vi "Read Value.vi"(8 "error in (no error)":errorcluster caption="entrée d'erreur (pas d'erreur)", 11 "DAQmxTaskAITension_Emulate en entrée":refnum<class "DAQmxTaskAIVoltage_Emulate.lvclass">) -> (0 "error out":errorcluster caption="sortie d'erreur", 1 "Data":bool, 2 "Data string":string, 3 "DAQmxTaskAITension_Emulate en sortie":refnum<class "DAQmxTaskAIVoltage_Emulate.lvclass">)   [LabVIEW 2018, in "DAQmxTaskAIVoltage_Emulate.lvclass"]
uses:
  DAQmxTaskAIVoltage_Emulate.lvclass
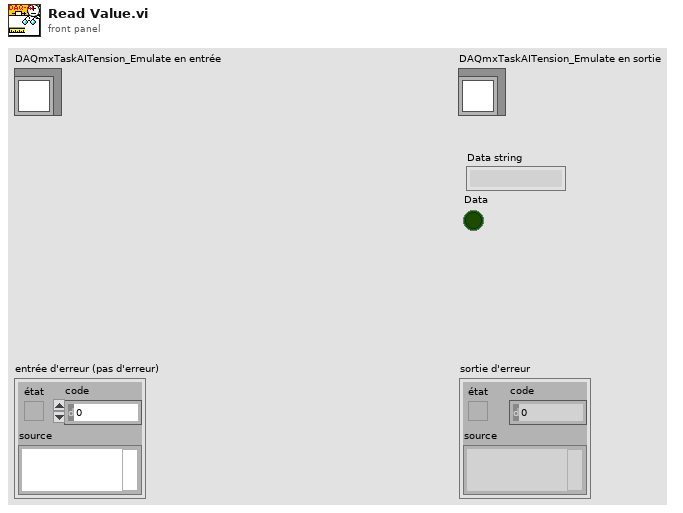
[diagram p1: front panel]
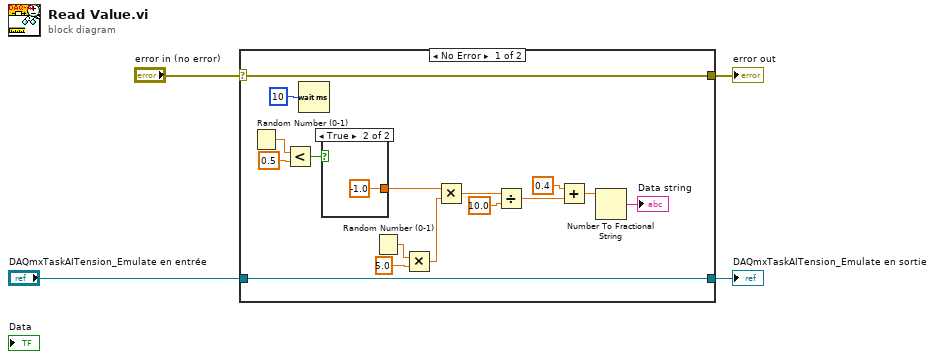
[diagram p0: block diagram]
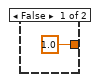
[diagram p2: hidden frame]
diagram:
  n1 = case shown="No Error" "error in (no error)" {
    selector: "error in (no error)" -> [w20 w24]
    tunnel: [w20 w24] -> w2
    tunnel: [w8 w23] -> w3
    tunnel: "DAQmxTaskAITension_Emulate en entrée" -> [w8 w23]
    frame No Error {
      n2 = Random Number (0-1)() -> (number: 0 to 1=w19:dbl)
      n3 = Less?(x=w19, y=0.5) -> (x < y?=w17:bool)
      n4 = Wait (ms)(milliseconds to wait=u32 10) -> ()  [unwired: 1 out]
      n5 = case shown="True" w17 {
        tunnel: [1.0 -1.0] -> w16
        frame False {
        }
        frame True {
        }
      }
      n6 = Random Number (0-1)() -> (number: 0 to 1=w15:dbl)
      n7 = Multiply(x=w15, y=5.0) -> (x*y=w13:dbl)
      n8 = Multiply(x=w16, y=w13) -> (x*y=w7:dbl)
      n9 = Divide(x=w7, y=10.0) -> (x/y=w5:dbl)
      n10 = Add(x=0.4, y=w5) -> (x+y=w11:dbl)
      n11 = Number To Fractional String(number=w11) -> (F-format string=→"Data string":string)  [unwired: 3 in]
    }
    frame Error {
    }
  }
  "error out" <- w2
  "DAQmxTaskAITension_Emulate en sortie" <- w3
